vi "Construct DMD 1 Image (SubVI).vi"(0 "DMD1X Array":dbl[][](array[numeric]), 5 "DMD1Y Array":dbl[][](array[numeric]), 6 "Stimulus Parameters":dbl[][](array[numeric]), 7 "DMD Intensity Cal Param":T1={"X2"=0.2142, "X1"=0.2142, "C"=0.2142}, 8 "Intensity Coefficients":dbl[][](array[numeric]), 10 "Pixel Resolution (um/Pixel)":dbl, 12 "Initialized DMD Image Array":dbl[][](array[numeric])) -> (14 "Image Array":u8[][](array[numeric]))   [LabVIEW 2020]
uses:
  Controls (HOST)/DMD Intensity Cal Param.ctl
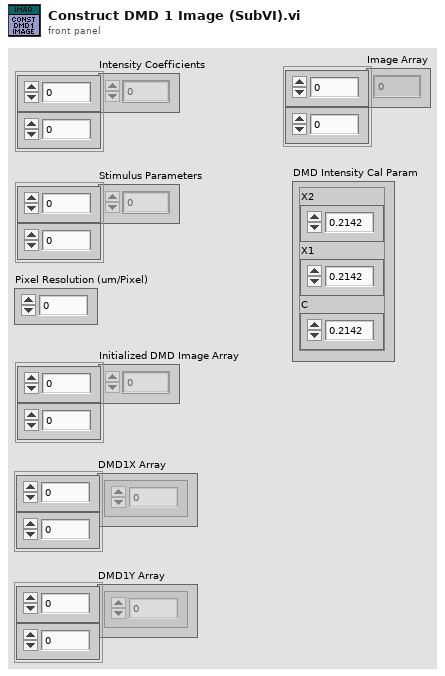
[diagram p1: front panel]
types:
  T1 = typedef "DMD Intensity Cal Param.ctl" = cluster{"X2":dbl, "X1":dbl, "C":dbl}
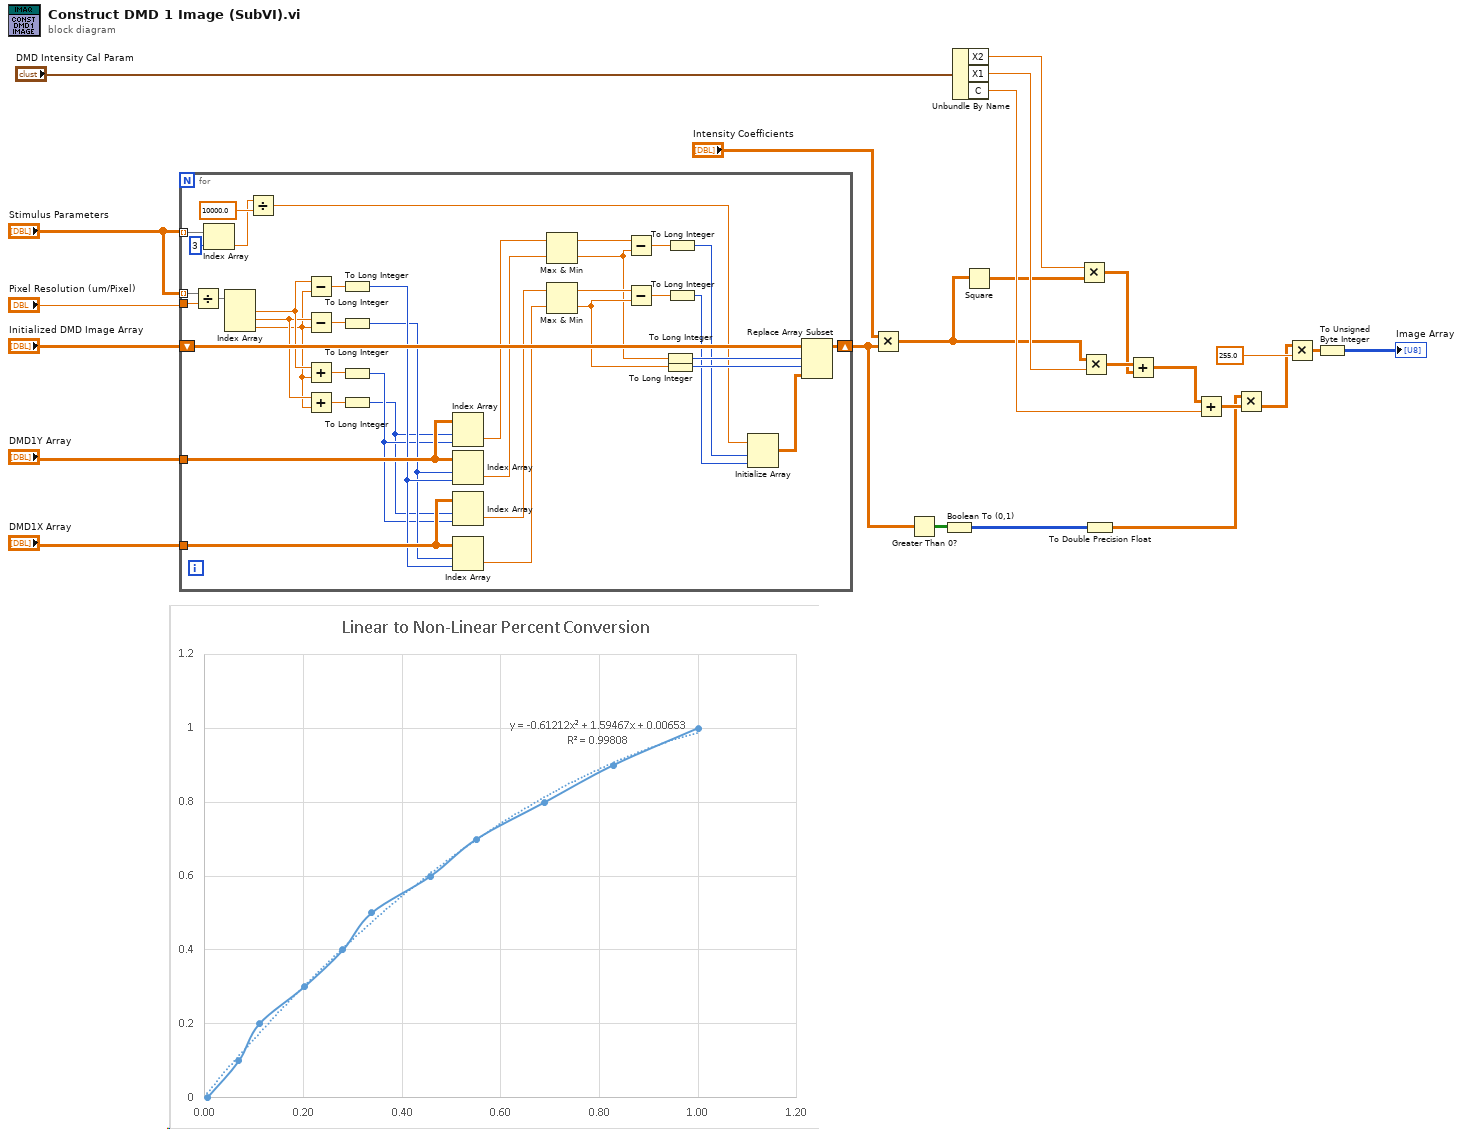
[diagram p0: block diagram]
diagram:
  n1 = for {
    shift-right: [w61] -> w18
    shift-left: "Initialized DMD Image Array" -> [w62]
    tunnel: "Stimulus Parameters" -> [w58] mode=indexing
    tunnel: "Pixel Resolution (um/Pixel)" -> [w56]
    tunnel: "Stimulus Parameters" -> [w55] mode=indexing
    tunnel: "DMD1Y Array" -> [w36]
    tunnel: "DMD1X Array" -> [w35]
    n2 = Divide(x=w58, y=w56) -> (x/y=w53:dbl[])
    n3 = Index Array(array=w55, index=3) -> (element=w25:dbl)
    n4 = Index Array(array=w53) -> (element #1=w42:dbl, element #2=w41:dbl, element #3=w34:dbl)  [unwired: 3 in]
    n5 = Divide(x=w25, y=10000.0) -> (x/y=w27:dbl)
    n6 = Subtract(x=w42, y=w34) -> (x-y=w38:dbl)
    n7 = Subtract(x=w41, y=w34) -> (x-y=w40:dbl)
    n8 = Add(x=w42, y=w34) -> (x+y=w37:dbl)
    n9 = Add(x=w41, y=w34) -> (x+y=w39:dbl)
    n10 = To Long Integer(number=w38) -> (32bit integer=w33:i32)
    n11 = To Long Integer(number=w40) -> (32bit integer=w32:i32)
    n12 = To Long Integer(number=w37) -> (32bit integer=w31:i32)
    n13 = To Long Integer(number=w39) -> (32bit integer=w30:i32)
    n14 = Index Array(array=w36, index (row)=w30, index (col)=w31) -> (element=w48:dbl)
    n15 = Index Array(array=w36, index (row)=w32, index (col)=w33) -> (element=w47:dbl)
    n16 = Index Array(array=w35, index (row)=w30, index (col)=w31) -> (element=w49:dbl)
    n17 = Index Array(array=w35, index (row)=w32, index (col)=w33) -> (element=w50:dbl)
    n18 = Max & Min(x=w48, y=w47) -> (max(x,y)=w44:dbl, min(x,y)=w28:dbl)
    n19 = Max & Min(x=w49, y=w50) -> (max(x,y)=w46:dbl, min(x,y)=w29:dbl)
    n20 = Subtract(x=w44, y=w28) -> (x-y=w43:dbl)
    n21 = Subtract(x=w46, y=w29) -> (x-y=w45:dbl)
    n22 = To Long Integer(number=w28) -> (32bit integer=w60:i32)
    n23 = To Long Integer(number=w29) -> (32bit integer=w59:i32)
    n24 = To Long Integer(number=w43) -> (32bit integer=w52:i32)
    n25 = To Long Integer(number=w45) -> (32bit integer=w51:i32)
    n26 = Initialize Array(w27, w52, w51) -> (w26:dbl[][])
    n27 = Replace Array Subset(array=w62, new element=w26, index (row)=w60, index (col)=w59) -> (w61:dbl[][])
  }
  n28 = Multiply(x="Intensity Coefficients", y=w18) -> (x*y=w9:dbl[][])
  n29 = Greater Than 0?(x=w18) -> (x > 0?=w4:bool[][])
  n30 = Boolean To (0,1)(Boolean=w4) -> (0, 1=w2:i16[][])
  n31 = Unbundle By Name("DMD Intensity Cal Param") -> ("X2"=w16:dbl, "X1"=w15:dbl, "C"=w14:dbl)
  n32 = Square(x=w9) -> (x^2=w10:dbl[][])
  n33 = Multiply(x=w16, y=w10) -> (x*y=w7:dbl[][])
  n34 = Multiply(x=w9, y=w15) -> (x*y=w8:dbl[][])
  n35 = To Double Precision Float(number=w2) -> (double precision float=w1:dbl[][])
  n36 = Add(x=w8, y=w7) -> (x+y=w6:dbl[][])
  n37 = Add(x=w6, y=w14) -> (x+y=w5:dbl[][])
  n38 = Multiply(x=w1, y=w5) -> (x*y=w3:dbl[][])
  n39 = Multiply(x=w3, y=255.0) -> (x*y=w12:dbl[][])
  n40 = To Unsigned Byte Integer(number=w12) -> (unsigned 8bit integer=→"Image Array":u8[][])
